vi "실습 1-3.vi"() -> ()   [LabVIEW 2014]
panel:
  out "x-y":u32
  in  "확인 버튼":bool
  out "웨이브폼 차트":dbl(graph)
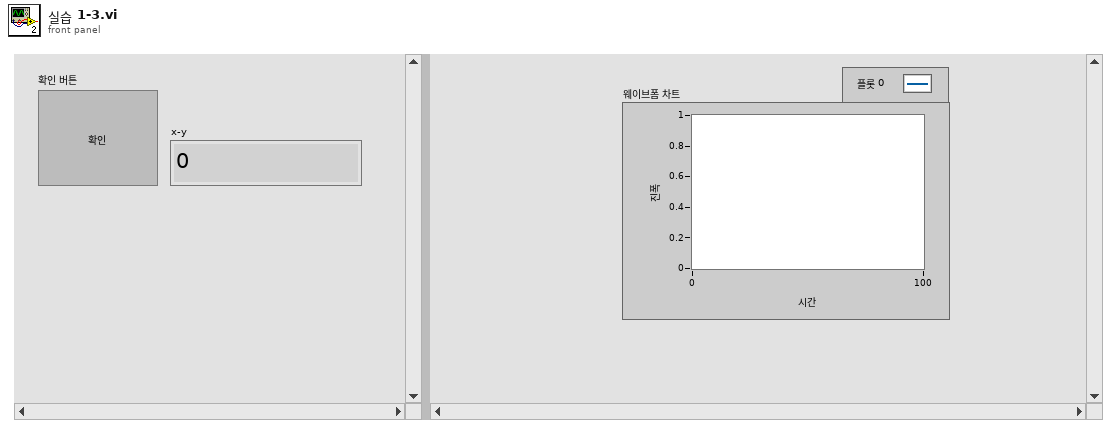
[diagram p1: front panel]
types:
  T1 = enum32{"invalid app kind", "Development System", "Run Time System", "Student Edition", "Embedded LabVIEW", "Evaluation", "Custom"}
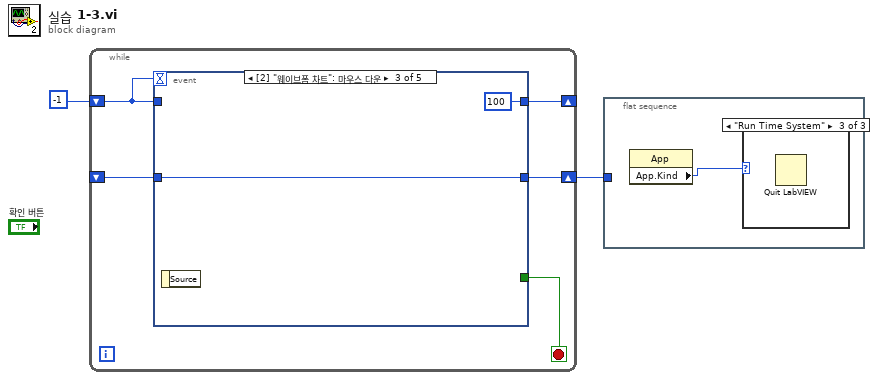
[diagram p0: block diagram]
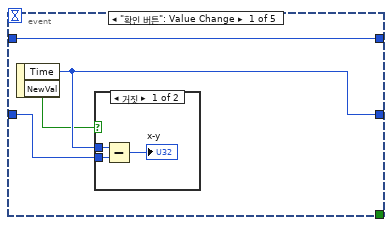
[diagram p4: hidden frame]
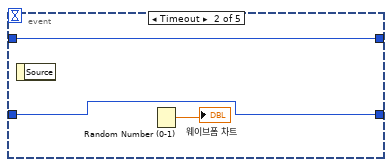
[diagram p6: hidden frame]
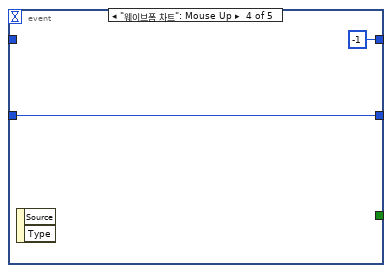
[diagram p7: hidden frame]
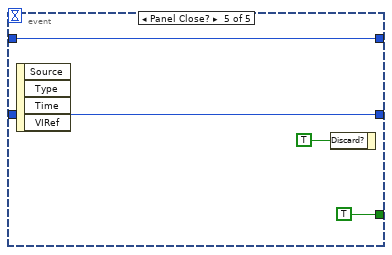
[diagram p8: hidden frame]
diagram:
  n1 = while {
    shift-right: [w6] -> w2
    shift-left: _ -> [w5]
    shift-right: [w3] -> _
    shift-left: -1 -> [w4]
    stop <- w7 stop-if-true
    n2 = event shown="[2] \"웨이브폼 차트\": 마우스 다운" {
      selector: _ -> [_ _ _ _ _]
      dyn-events: _ -> [_ _ _ _ _]
      timeout: w4 -> [_ _ _ _ _]
      tunnel: [_ _ _ _ TRUE] -> w7
      tunnel: [w11 w15 w18 w20 w22] -> w6
      tunnel: w5 -> [w10 w15 w18 w20 w22]
      tunnel: w4 -> [w8 w16 _ _ w23]
      tunnel: [w8 w16 100 -1 w23] -> w3
      event "확인 버튼": Value Change {
        n3 = event-data() -> ("Time"=w11:u32, "NewVal"=w9:bool)  [unwired: 1 in]
        n4 = case shown="거짓" w9 {
          tunnel: w11 -> [w14 _]
          tunnel: w10 -> [w13 _]
          frame False {
            n5 = Subtract(x=w14, y=w13) -> (x-y=→"x-y":u32)
          }
          frame True {
          }
        }
      }
      event Timeout {
        n6 = event-data() -> ()  [unwired: 1 in, 1 out]
        n7 = Random Number (0-1)() -> (number: 0 to 1=→"웨이브폼 차트":dbl)
      }
      event "웨이브폼 차트": Mouse Down {
        n8 = event-data() -> ()  [unwired: 1 in, 1 out]
      }
      event "웨이브폼 차트": Mouse Up {
        n9 = event-data() -> ()  [unwired: 1 in, 2 out]
      }
      event Panel Close? {
        n10 = event-data() -> ()  [unwired: 1 in, 4 out]
        n11 = event-data("Discard?"=TRUE) -> ()  [unwired: 1 in, 1 out]
      }
    }
  }
  n12 = flat-sequence {
    tunnel: w2 -> [_]
    frame #0 {
      n13 = property class="App"() -> ("App.Kind"=w26:T1)  [unwired: 2 in, 2 out]
      n14 = case shown="\"Run Time System\"" w26 {
        frame "invalid app kind", Default {
        }
        frame "Development System" {
        }
        frame "Run Time System" {
          n15 = Quit LabVIEW() -> ()  [unwired: 1 in]
        }
      }
    }
  }
